vi "Measured.vi"(8 "error in (no error)":errorcluster, 11 "CodeCoverage in":refnum<class "CodeCoverage.lvclass">) -> (0 "error out":errorcluster, 2 "All VIs Measured":path[](array[path]), 3 "CodeCoverage out":refnum<class "CodeCoverage.lvclass">)   [LabVIEW 2019, in "CodeCoverage.lvclass"]
uses:
  CodeCoverage.lvclass
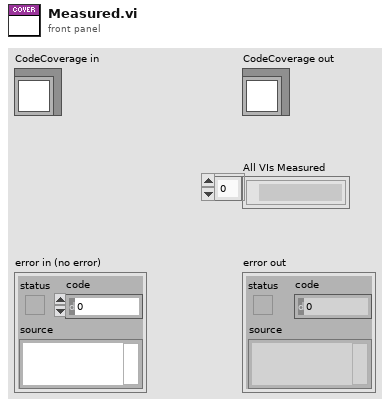
[diagram p1: front panel]
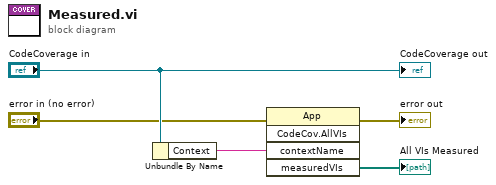
[diagram p0: block diagram]
diagram:
  n1 = Unbundle By Name("CodeCoverage in") -> ("Context"=w4:string)
  n2 = invoke class="App" method="CodeCov.AllVIs"(error in="error in (no error)", "contextName"=w4) -> (error out=→"error out":errorcluster, "measuredVIs"=→"All VIs Measured":path[])  [unwired: 3 in, 3 out]
  "CodeCoverage out" <- "CodeCoverage in"
